vi "Field Draw Field.vi"(6 "Lado,radius, stretch":i32[](array[numeric]), 8 "new picture in":picture, 9 "Offset":cluster{"Width":dbl, "Height":dbl}, 10 "Scale":dbl, 11 "Field Size in":T1) -> (0 "new picture out":picture, 1 "Offset Out":cluster{"Width":dbl, "Height":dbl}, 2 "Scale Out":dbl)   [LabVIEW 2018]
panel:
  in  "left":i16=1
  in  "rect":T2
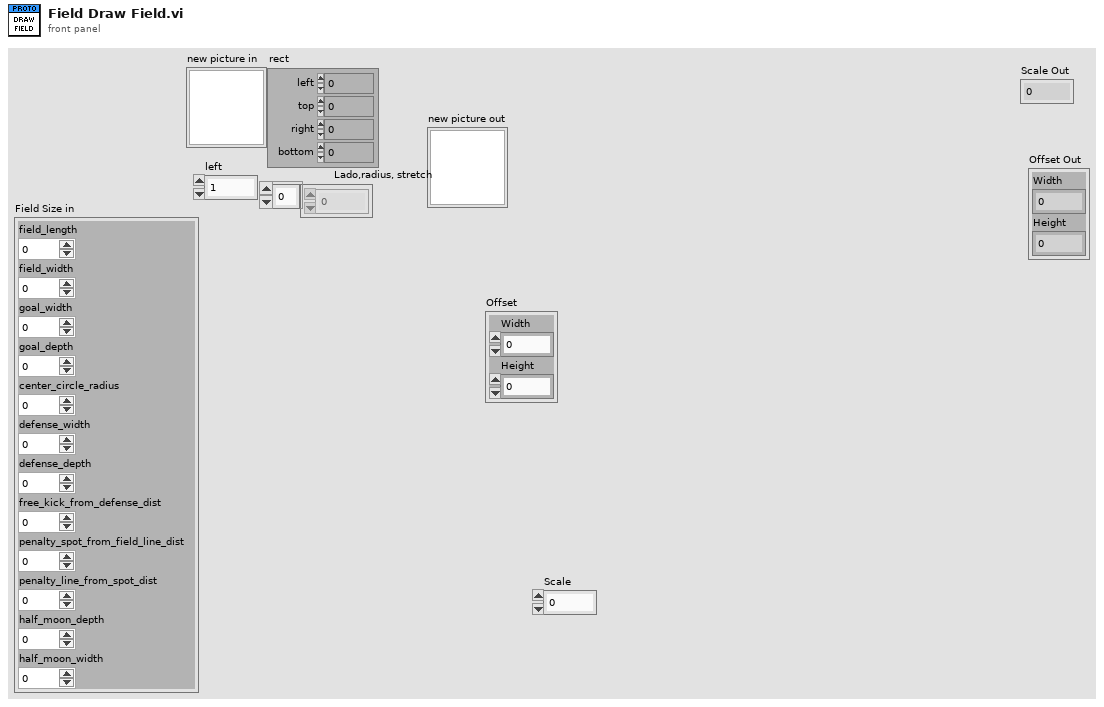
[diagram p1: front panel]
types:
  T1 = cluster{"field_length":u32, "field_width":u32, "goal_width":u32, "goal_depth":u32, "center_circle_radius":u32, "defense_width":u32, "defense_depth":u32, "free_kick_from_defense_dist":u32, "penalty_spot_from_field_line_dist":u32, "penalty_line_from_spot_dist":u32, "half_moon_depth":u32, "half_moon_width":u32}
  T2 = cluster{"left":i16, "top":i16, "right":i16, "bottom":i16}
  T3 = cluster{"Width":i16, "Style":enum32{"Solid", "Dash", "Dot", "DashDot", "DashDotDot"}}
  T4 = cluster{"field_length":dbl, "field_width":dbl, "goal_width":dbl, "goal_depth":dbl, "center_circle_radius":dbl, "defense_width":dbl, "defense_depth":dbl, "free_kick_from_defense_dist":dbl, "penalty_spot_from_field_line_dist":dbl, "penalty_line_from_spot_dist":dbl, "half_moon_depth":dbl, "half_moon_width":dbl}
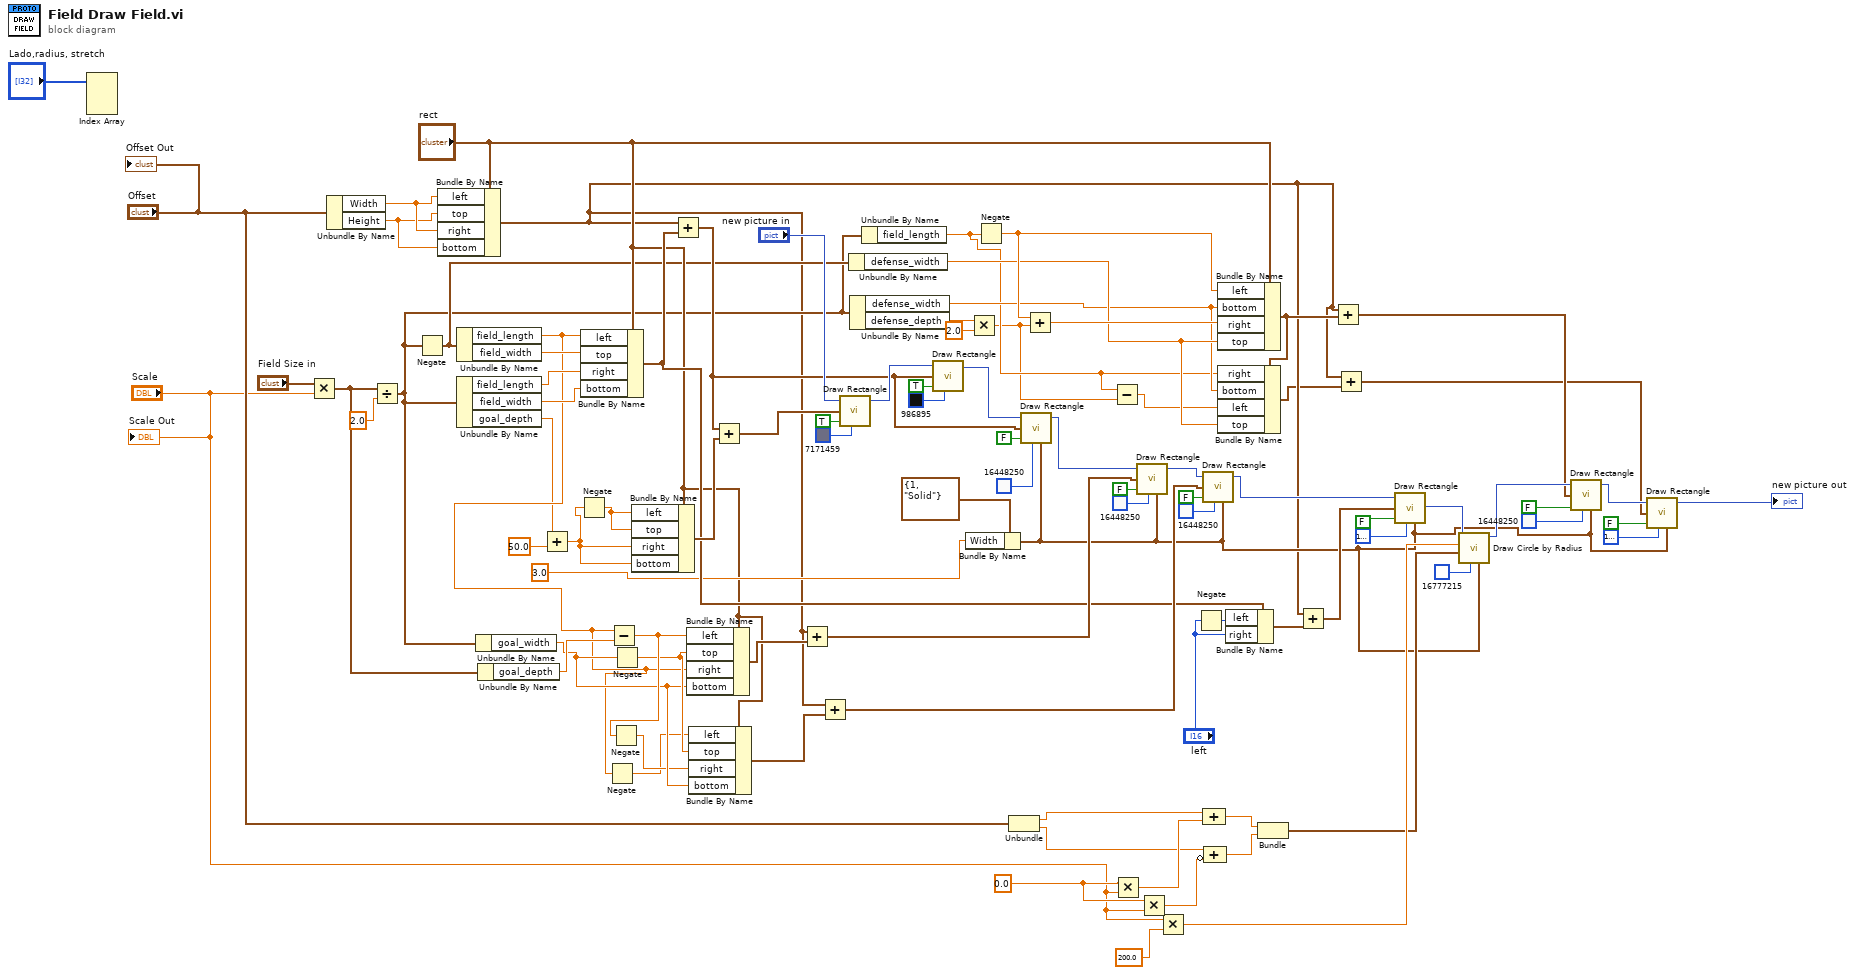
[diagram p0: block diagram]
diagram:
  w37 = 0.0 ("x")
  n1 = Index Array(array="Lado,radius, stretch") -> ()  [unwired: 3 in, 3 out]
  n2 = Multiply(x="Field Size in", y="Scale") -> (x*y=w36:T4)
  n3 = Unbundle By Name("Offset") -> ("Width"=w88:dbl, "Height"=w87:dbl)
  n4 = Divide(x=w36, y=2.0) -> (x/y=w20:T4)
  n5 = Negate(x=w20) -> (-x=w21:T4)
  n6 = Bundle By Name(cluster="rect", "left"=w88, "top"=w87, "right"=w88, "bottom"=w87) -> (w3:T2)
  n7 = Unbundle By Name(w21) -> ("field_length"=w32:dbl, "field_width"=w86:dbl)
  n8 = Unbundle By Name(w20) -> ("field_length"=w85:dbl, "field_width"=w84:dbl, "goal_depth"=w27:dbl)
  n9 = Unbundle By Name(w20) -> ("goal_width"=w61:dbl)
  n10 = Unbundle By Name(w36) -> ("goal_depth"=w66:dbl)
  n11 = Add(x=w27, y=50.0) -> (x+y=w28:dbl)
  n12 = Negate(x=w28) -> (-x=w83:dbl)
  n13 = Bundle By Name(cluster="rect", "left"=w32, "top"=w86, "right"=w85, "bottom"=w84) -> (w54:T2)
  n14 = Negate(x=w32) -> (-x=w57:dbl)
  n15 = Subtract(x=w32, y=w66) -> (x-y=w63:dbl)
  n16 = Negate(x=w63) -> (-x=w58:dbl)
  n17 = Negate(x=w61) -> (-x=w62:dbl)
  n18 = Bundle By Name(cluster="rect", "left"=w83, "top"=w83, "right"=w28, "bottom"=w28) -> (w82:T2)
  n19 = Add(x=w3, y=w54) -> (x+y=w47:T2)
  n20 = Bundle By Name(cluster="rect", "left"=w63, "top"=w62, "right"=w32, "bottom"=w61) -> (w65:T2)
  n21 = Bundle By Name(cluster="rect", "left"=w57, "top"=w62, "right"=w58, "bottom"=w61) -> (w60:T2)
  n22 = Add(x=w47, y=w82) -> (x+y=w78:T2)
  n23 = Add(x=w3, y=w65) -> (x+y=w64:T2)
  n24 = Add(x=w3, y=w60) -> (x+y=w59:T2)
  n25 = call <vilib>:"Draw Rectangle.vi"("picture"="new picture in", "rect"=w78, "fill?(F)"=TRUE, "color(black)"=u32 7171459) -> ("new picture"=w77:picture)  [unwired: 5 in]
  n26 = Unbundle By Name(w21) -> ("defense_width"=w8:dbl)
  n27 = Unbundle By Name(w20) -> ("defense_width"=w7:dbl, "defense_depth"=w14:dbl)
  n28 = Unbundle By Name(w20) -> ("field_length"=w6:dbl)
  n29 = call <vilib>:"Draw Rectangle.vi"("picture"=w77, "rect"=w47, "fill?(F)"=TRUE, "color(black)"=u32 986895) -> ("new picture"=w74:picture)  [unwired: 5 in]
  n30 = Bundle By Name(cluster=T3 {"Width"=1, "Style"=enum."Solid"} ("pen"), "Width"=3.0) -> (w11:T3)
  n31 = Multiply(x=w14, y=2.0) -> (x*y=w5:dbl)
  n32 = Negate(x=w6) -> (-x=w15:dbl)
  n33 = Unbundle("Offset") -> ("Width"=w45:dbl, "Height"=w42:dbl)
  n34 = call <vilib>:"Draw Rectangle.vi"("picture"=w74, "rect"=w47, "fill?(F)"=FALSE, "color(black)"=u32 16448250, "pen"=w11) -> ("new picture"=w70:picture)  [unwired: 4 in]
  n35 = Add(x=w15, y=w5) -> (x+y=w12:dbl)
  n36 = Subtract(x=w6, y=w5) -> (x-y=w4:dbl)
  n37 = Multiply(x=w37, y="Scale") -> (x*y=w44:dbl)
  n38 = call <vilib>:"Draw Rectangle.vi"("picture"=w70, "rect"=w64, "fill?(F)"=FALSE, "color(black)"=u32 16448250, "pen"=w11) -> ("new picture"=w67:picture)  [unwired: 4 in]
  n39 = Multiply(x=w37, y="Scale") -> (x*y=w41:dbl)
  n40 = Multiply(x="Scale", y=sgl 200.0 ("radius")) -> (x*y=w39:dbl)
  n41 = Negate(x="left") -> (-x=w50:i16)
  n42 = call <vilib>:"Draw Rectangle.vi"("picture"=w67, "rect"=w59, "fill?(F)"=FALSE, "color(black)"=u32 16448250, "pen"=w11) -> ("new picture"=w30:picture)  [unwired: 4 in]
  n43 = Compound Arithmetic op=ADD(w45, w44) -> (w43:dbl)
  n44 = Compound Arithmetic op=ADD(w42, invert w41) -> (w40:dbl)
  n45 = Bundle By Name(cluster="rect", "left"=w15, "bottom"=w7, "right"=w12, "top"=w8) -> (w9:T2)
  n46 = Bundle By Name(cluster=w9, "right"=w6, "bottom"=w7, "left"=w4, "top"=w8) -> (w2:T2)
  n47 = Bundle By Name(cluster=w54, "left"=w50, "right"="left") -> (w53:T2)
  n48 = Bundle(w43, w40) -> (w38:cluster{dbl, dbl})  [unwired: 1 in]
  n49 = Add(x=w3, y=w53) -> (x+y=w52:T2)
  n50 = Add(x=w3, y=w9) -> (x+y=w10:T2)
  n51 = Add(x=w3, y=w2) -> (x+y=w1:T2)
  n52 = call <vilib>:"Draw Rectangle.vi"("picture"=w30, "rect"=w52, "fill?(F)"=FALSE, "color(black)"=u32 16777226, "pen"=w11) -> ("new picture"=w49:picture)  [unwired: 4 in]
  n53 = call <vilib>:"Draw Circle by Radius.vi"("pen"=w11, "color(black)"=u32 16777215, "pixel center"=w38, "radius"=w39, "picture"=w49) -> ("new picture"=w25:picture)  [unwired: 6 in]
  n54 = call <vilib>:"Draw Rectangle.vi"("picture"=w25, "rect"=w10, "fill?(F)"=FALSE, "color(black)"=u32 16448250, "pen"=w11) -> ("new picture"=w19:picture)  [unwired: 4 in]
  n55 = call <vilib>:"Draw Rectangle.vi"("picture"=w19, "rect"=w1, "fill?(F)"=FALSE, "color(black)"=u32 16777226, "pen"=w11) -> ("new picture"=→"new picture out":picture)  [unwired: 4 in]
  "Scale Out" <- "Scale"
  "Offset Out" <- "Offset"
